vi "FRA_sensors_main.vi"() -> ()   [LabVIEW 2013]
uses:
  subVIs/UDP_read_datagram.ctl
  subVIs/UI_states.ctl
  <vilib>/Utility/file.llb/Read From Spreadsheet File (string).vi
panel:
  out "ACK'd_clients addr":u32[](array[numeric]) format="%x"
  in  "Power all sensors":bool
  out "Number of clients":i32
  in  "OK Button":bool
  in  "Power A3.3":bool
  in  "Power A3.2":bool
  in  "Power A3.1":bool
  in  "Power A3.0":bool
  in  "Power A2.3":bool
  in  "Power A2.2":bool
  in  "Power A2.1":bool
  in  "Power A2.0":bool
  in  "Power A1.3":bool
  in  "Power A1.2":bool
  in  "Power A1.1":bool
  in  "Power A1.0":bool
  out "Error message":string
  in  "listen on port":u16=1100
  out "data received":string
  in  "Stop Button":bool
  out "Datagram to send":string
  out "ACK'd_clients":u8[](array[numeric])
  # "OFF"
  # "ON"
  # "variables and settings"
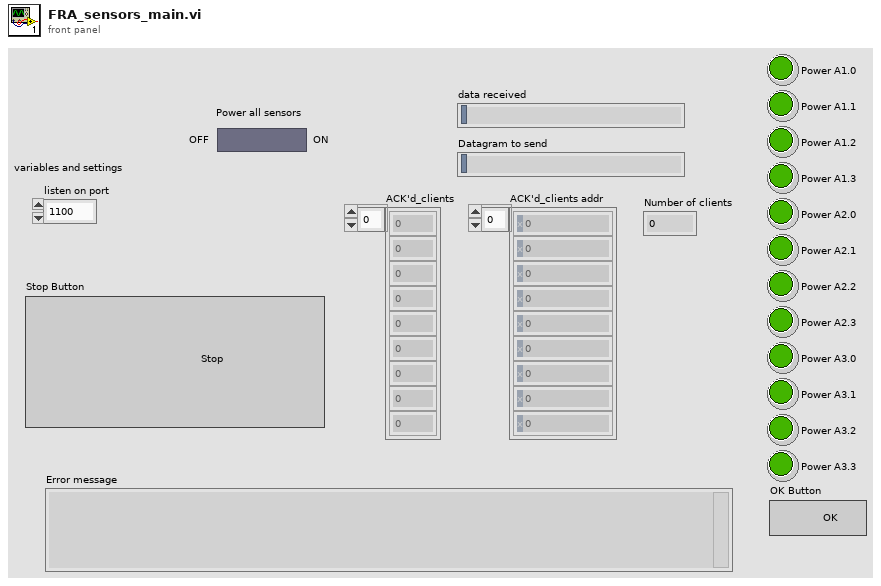
[diagram p1: front panel]
types:
  T1 = typedef "UI_states.ctl" = enum16{"SENS_PWR_CHANGE", "INIT", "IDLE", "RUN", "STOP", ""}
  T2 = typedef "UDP_read_datagram.ctl" = cluster{"msg":string, "address":u32, "port":u16}
  T3 = enum8{"Enabled", "Disabled", "Disabled and Grayed Out"}
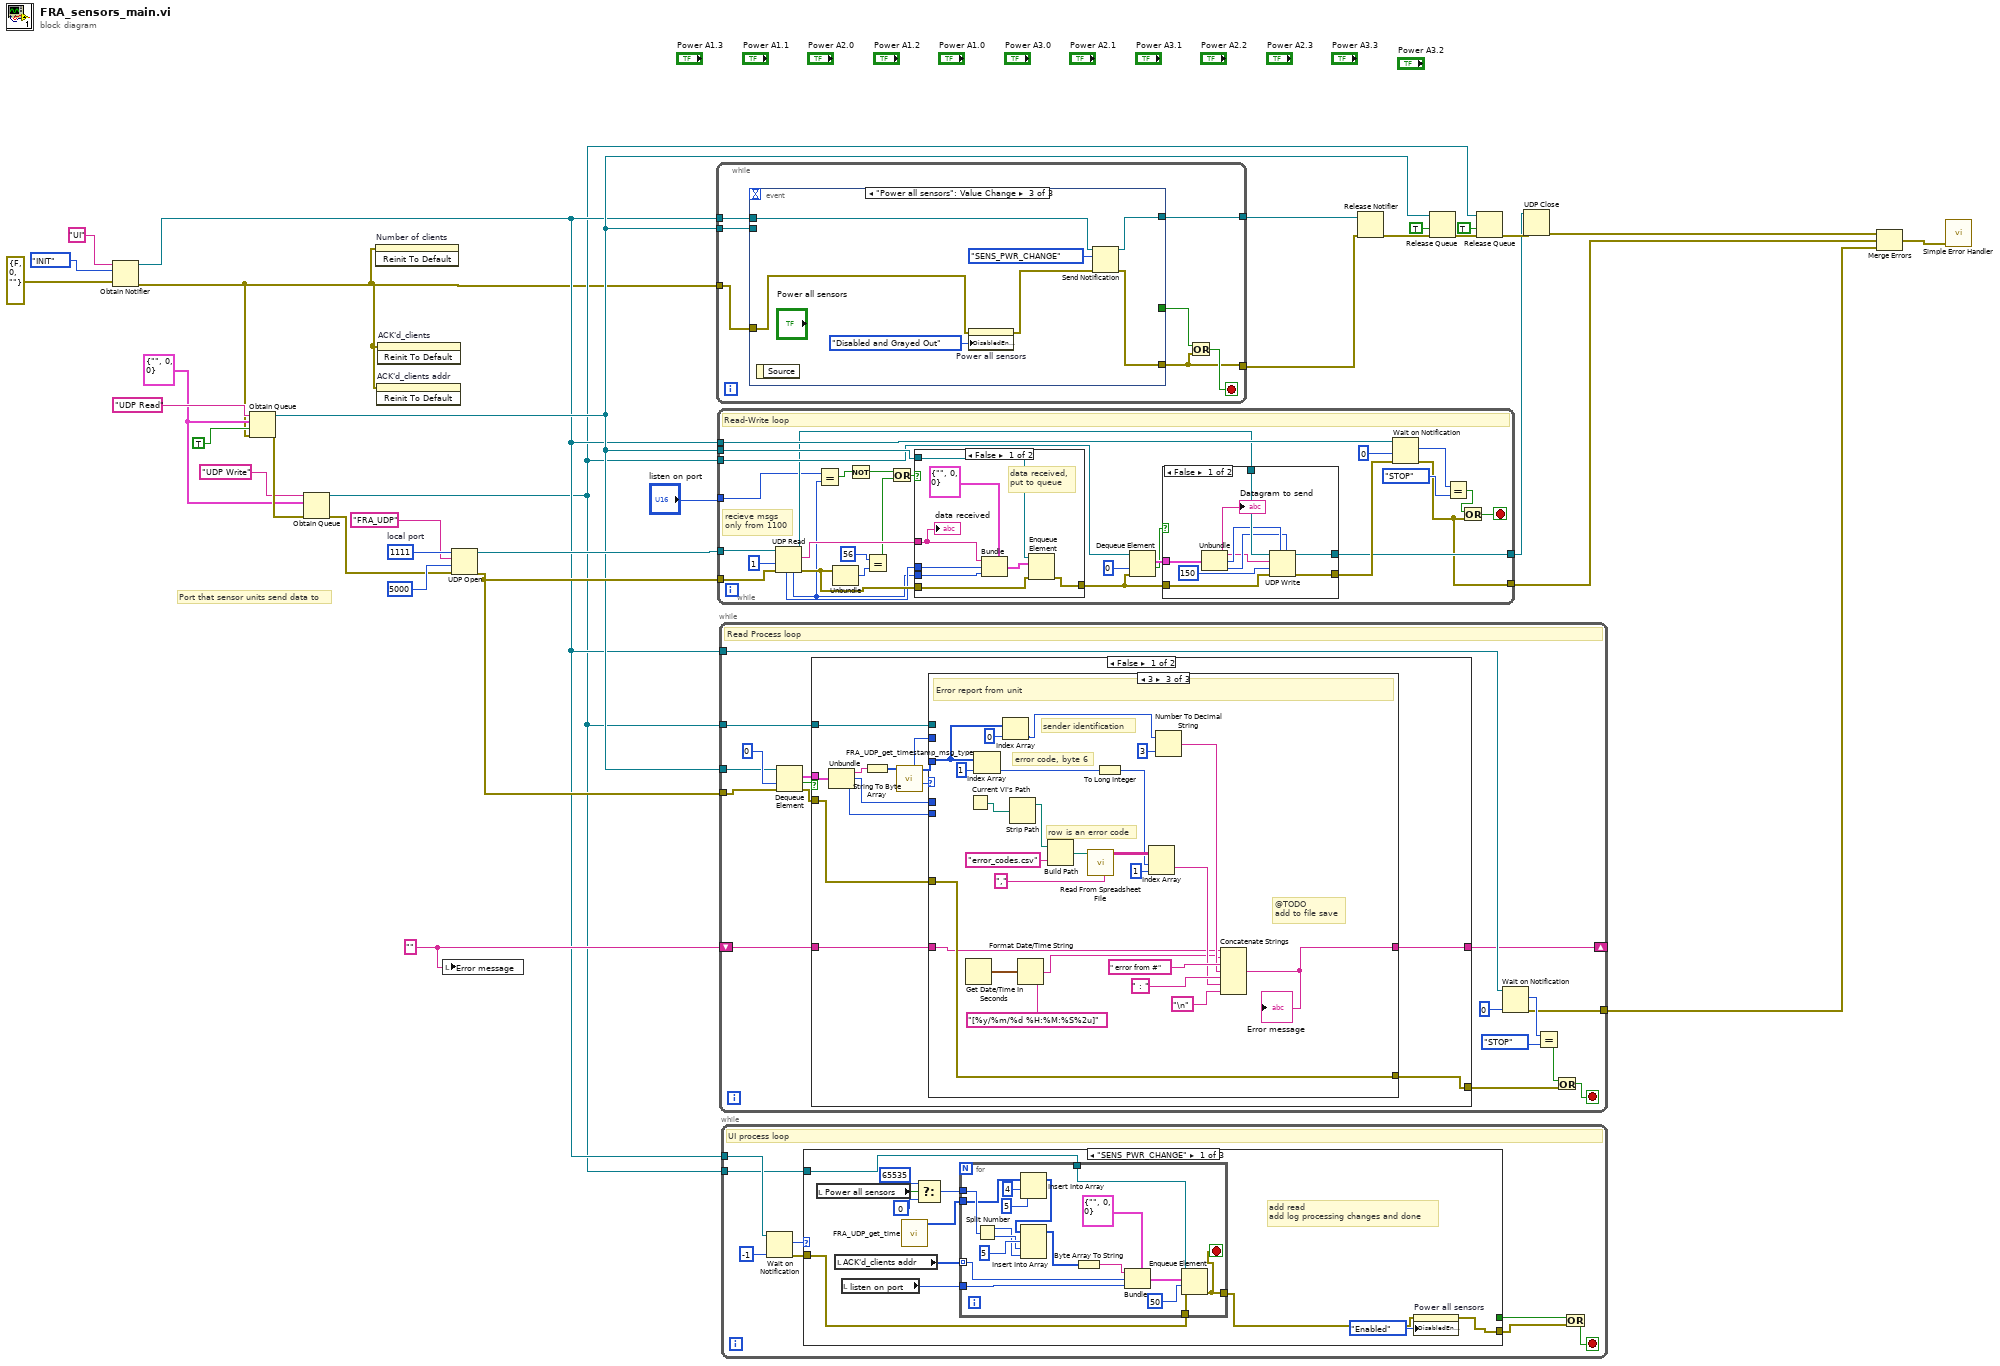
[diagram p0: block diagram]
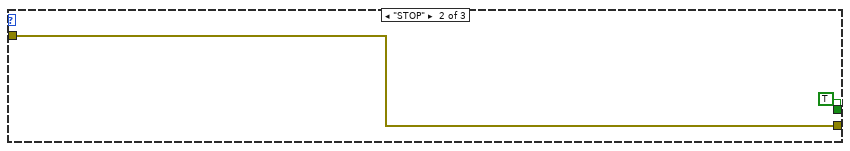
[diagram p2: hidden frame]
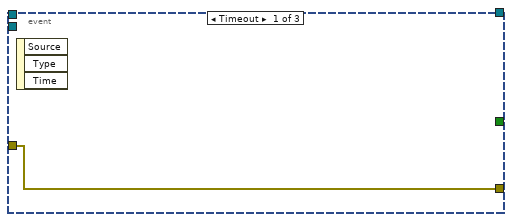
[diagram p4: hidden frame]
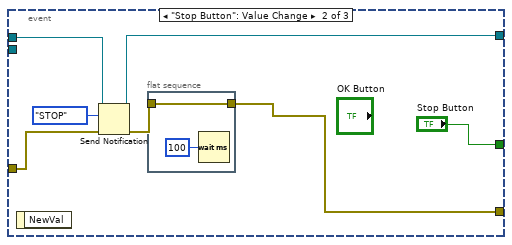
[diagram p5: hidden frame]
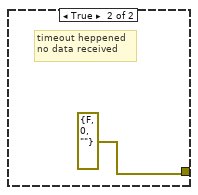
[diagram p7: hidden frame]
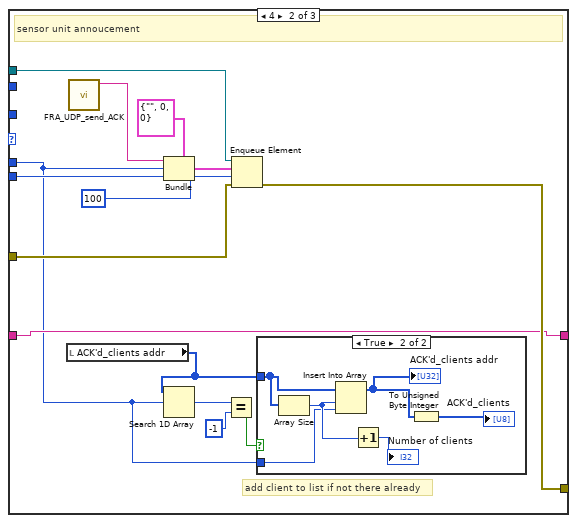
[diagram p9: hidden frame]
diagram:
  w4 = ""
  w13 = T2 {"msg"="", "address"=0, "port"=0}
  w32 = u16 1111  # local port
  # "Port that sensor units send data to"
  n1 = Obtain Notifier(name (unnamed)="UI", notification data type=UI_states."INIT" ("Enum"), error in (no error)=errorcluster {"status"=FALSE, "code"=0, "source"=""}) -> (notifier out=w3:refnum<notifier>, error out=w1:errorcluster)  [unwired: 1 in, 1 out]
  n2 = Obtain Queue(name (unnamed)="UDP Read", element data type=w13, create if not found? (T)=TRUE, error in (no error)=w1) -> (queue out=w9:refnum<queue>, error out=w15:errorcluster)  [unwired: 1 in, 1 out]
  n3 = Obtain Queue(name (unnamed)="UDP Write", element data type=w13, error in (no error)=w15) -> (queue out=w2:refnum<queue>, error out=w12:errorcluster)  [unwired: 2 in, 1 out]
  n4 = invoke on="Number of clients" class="DigNum (strict)" method="Reinit To Default"(error in=w1) -> ()  [unwired: 2 in, 3 out]
  n5 = invoke on="ACK'd_clients addr" class="Arr (strict)" method="Reinit To Default"(error in=w1) -> ()  [unwired: 2 in, 3 out]
  n6 = invoke on="ACK'd_clients" class="Arr (strict)" method="Reinit To Default"(error in=w1) -> ()  [unwired: 2 in, 3 out]
  n7 = local write "Error message"(w4) -> ()
  n8 = UDP Open(8:w12, 9:5000 ("timeout ms (25000)"), 10:"FRA_UDP" ("service name"), 11:w32) -> (port=w26:refnum<k16>, 0:w27:errorcluster)  [unwired: 1 in, 1 out]
  n9 = while {
    tunnel: w3 -> [w39]
    tunnel: w1 -> [w38]
    tunnel: [w35] -> w22
    tunnel: [w34] -> w21
    tunnel: w9 -> [w33]
    stop <- w36 stop-if-true
    n10 = event shown="[2] \"Power all sensors\": Value Change" {
      selector: _ -> [_ _ _]
      dyn-events: _ -> [_ _ _]
      timeout: _ -> [_ _ _]
      tunnel: w39 -> [_ w46 w55]
      tunnel: [w40 w41 w50] -> w34
      tunnel: w38 -> [w40 w44 w52]
      tunnel: [_ "Stop Button" _] -> w37
      tunnel: [_ w43 w54] -> w35
      tunnel: w33 -> [_ _ _]
      event Timeout {
        n11 = event-data() -> ()  [unwired: 1 in, 3 out]
      }
      event "Stop Button": Value Change {
        n12 = event-data() -> ()  [unwired: 1 in, 1 out]
        n13 = Send Notification(notification=UI_states."STOP", notifier=w46, error in (no error)=w44) -> (notifier out=w43:refnum<notifier>, error out=w42:errorcluster)
        n14 = flat-sequence {
          tunnel: w42 -> [w48]
          tunnel: [w48] -> w41
          frame #0 {
            n15 = Wait (ms)(milliseconds to wait=u32 100) -> ()  [unwired: 1 out]
          }
        }
      }
      event "Power all sensors": Value Change {
        n16 = event-data() -> ()  [unwired: 1 in, 1 out]
        n17 = property on="Power all sensors" class="Bool (strict)"(error in=w52, "DisabledEnum"=T3."Disabled and Grayed Out" ("Disabled")) -> (error out=w51:errorcluster)  [unwired: 1 in, 1 out]
        n18 = Send Notification(notification=UI_states."SENS_PWR_CHANGE", notifier=w55, error in (no error)=w51) -> (notifier out=w54:refnum<notifier>, error out=w50:errorcluster)
      }
    }
    n19 = Or(x=w37, y=w34) -> (x .or. y?=w36:bool)
  }
  n20 = while {
    tunnel: w9 -> [w75]
    tunnel: w27 -> [w80]
    tunnel: w26 -> [w85]
    tunnel: w3 -> [w84]
    tunnel: w2 -> [w72]
    tunnel: [w61] -> w11
    tunnel: "listen on port" -> [w60]
    tunnel: [w57] -> w8
    stop <- w58 stop-if-true
    # "recieve msgs\nonly from 1100"
    # "Read-Write loop"
    n21 = UDP Read(connection ID=w85, timeout ms (25000)=1, 8:w80) -> (data out=w76:string, error out=w77:errorcluster, 3:w70:refnum<k16>, 4:w63:u16, 6:w74:u32)  [unwired: 1 out]
    n22 = Equal?(x=w60, y=w63) -> (x = y?=w65:bool)
    n23 = Unbundle(w77) -> ("code"=w79:i32)  [unwired: 2 out]
    n24 = Not(x=w65) -> (.not. x?=w64:bool)
    n25 = Equal?(x=56, y=w79) -> (x = y?=w66:bool)
    n26 = Or(x=w64, y=w66) -> (x .or. y?=w67:bool)
    n27 = case shown="False" w67 {
      tunnel: w77 -> [w105 _]
      tunnel: [w99 errorcluster {"status"=FALSE, "code"=0, "source"=""} ("error out")] -> w69
      tunnel: w76 -> [w102 _]
      tunnel: w75 -> [w98 _]
      tunnel: w74 -> [w101 _]
      tunnel: w63 -> [w100 _]
      frame False {
        # "data received, \nput to queue"
        n28 = Bundle(cluster=T2 {"msg"="", "address"=0, "port"=0}, "msg"=w102, "address"=w101, "port"=w100) -> (w104:T2)
        n29 = Enqueue Element(queue=w98, element=w104, error in (no error)=w105) -> (error out=w99:errorcluster)  [unwired: 1 in, 2 out]
        "data received" <- w102
      }
      frame True {
        # "timeout heppened\nno data received"
      }
    }
    n30 = Dequeue Element(queue=w72, timeout in ms (-1)=0, error in (no error)=w69) -> (element=w71:T2, timed out?=w62:bool)  [unwired: 2 out]
    n31 = case shown="False" w62 {
      tunnel: w71 -> [w95 _]
      tunnel: w70 -> [w94 w96]
      tunnel: w69 -> [w92 w97]
      tunnel: [w89 w97] -> w68
      tunnel: [w88 w96] -> w61
      frame False {
        n32 = Unbundle(w95) -> ("msg"=w87:string, "address"=w91:u32, "port"=w90:u16)
        "Datagram to send" <- w87
        n33 = UDP Write(address=w91, port or service name=w90, connection ID=w94, data in=w87, 8:w92, 9:150 ("timeout ms (25000)")) -> (error out=w89:errorcluster, 3:w88:refnum<k16>)
      }
      frame True {
        # "no message in send buffer"
      }
    }
    n34 = Wait on Notification(notifier=w84, timeout in ms (-1)=0, error in (no error)=w68) -> (notification=w82:T1, error out=w57:errorcluster)  [unwired: 1 in, 2 out]
    n35 = Equal?(x=w82, y=UI_states."STOP") -> (x = y?=w59:bool)
    n36 = Or(x=w59, y=w57) -> (x .or. y?=w58:bool)
  }
  n37 = while {
    tunnel: w27 -> [w122]
    tunnel: w9 -> [w121]
    tunnel: w3 -> [w111]
    tunnel: w2 -> [w109]
    tunnel: [w110] -> w7
    shift-right: [w107] -> _
    shift-left: w4 -> [w108]
    stop <- w116 stop-if-true
    # "Read Process loop"
    n38 = Dequeue Element(queue=w121, timeout in ms (-1)=0, error in (no error)=w122) -> (element=w118:T2, timed out?=w120:bool, error out=w119:errorcluster)  [unwired: 1 out]
    n39 = case shown="False" w120 {
      tunnel: w119 -> [w127 w185]
      tunnel: w118 -> [w134 _]
      tunnel: [w126 w185] -> w117
      tunnel: w109 -> [w129 _]
      tunnel: w108 -> [w125 w184]
      tunnel: [w124 w184] -> w107
      frame False {
        n40 = Unbundle(w134) -> ("msg"=w133:string, "address"=w130:u32, "port"=w128:u16)
        n41 = String To Byte Array(string=w133) -> (unsigned byte array=w136:u8[])
        n42 = call "FRA_UDP_get_timestamp_msg_type.vi"("incoming_UDP"=w136) -> ("MSG_type_byte"=w135:u8, "datagram_rest"=w132:u8[], "Datagram number"=w131:u32)  [unwired: 6 in, 2 out]
        n43 = case shown="3" w135 {
          tunnel: w132 -> [_ _ w160]
          tunnel: w131 -> [_ _ _]
          tunnel: w130 -> [_ w140 _]
          tunnel: w129 -> [_ w145 _]
          tunnel: w128 -> [_ w147 _]
          tunnel: w127 -> [w138 w143 w171]
          tunnel: [w138 w142 w171] -> w126
          tunnel: w125 -> [w137 w141 w166]
          tunnel: [w137 w141 w169] -> w124
          frame 0, Default {
          }
          frame 4 {
            # "add client to list if not there already"
            # "sensor unit annoucement"
            n44 = local read "ACK'd_clients addr"() -> (w139:u32[])
            n45 = call "FRA_UDP_send_ACK.vi"() -> ("Datagram to send"=w148:string)  [unwired: 11 in]
            n46 = Bundle(cluster=T2 {"msg"="", "address"=0, "port"=0}, "msg"=w148, "address"=w140, "port"=w147) -> (w146:T2)
            n47 = Search 1D Array(1D array=w139, element=w140) -> (index of element=w152:i32)  [unwired: 1 in]
            n48 = Equal?(x=w152, y=-1) -> (x = y?=w150:bool)
            n49 = Enqueue Element(queue=w145, element=w146, timeout in ms (-1)=100, error in (no error)=w143) -> (error out=w142:errorcluster)  [unwired: 2 out]
            n50 = case shown="True" w150 {
              tunnel: w139 -> [_ w158]
              tunnel: w140 -> [_ w156]
              frame False {
              }
              frame True {
                n51 = Array Size(array=w158) -> (size(s)=w157:i32)
                n52 = Insert Into Array(array=w158, index=w157, new element=w156) -> (w153:u32[])
                "ACK'd_clients addr" <- w153
                n53 = Increment(x=w157) -> (x+1=→"Number of clients":i32)
                n54 = To Unsigned Byte Integer(number=w153) -> (unsigned 8bit integer=→"ACK'd_clients":u8[])
              }
            }
          }
          frame 3 {
            # "sender identification"
            # "error code, byte 6"
            # "@TODO\nadd to file save"
            # "row is an error code"
            # "Error report from unit"
            n55 = Get Date/Time In Seconds() -> (seconds since 1Jan1904=w165:timestamp)
            n56 = Current VI's Path() -> (path=w168:path)
            n57 = Index Array(array=w160, index=1) -> (element=w177:u8)
            n58 = Index Array(array=w160, index=0) -> (element=w159:u8)
            n59 = Strip Path(path=w168) -> (stripped path=w167:path)  [unwired: 1 out]
            n60 = Format Date/Time String(time format string (%c)="[%y/%m/%d %H:%M:%S%2u]", seconds (now)=w165) -> (date/time string=w164:string)  [unwired: 1 in]
            n61 = Build Path(base path=w167, name or relative path="error_codes.csv") -> (appended path=w182:path)
            n62 = call-poly <vilib>:"Read From Spreadsheet File.vi"("delimiter (\\t)"="," ("delimiter (\\t)"), "file path (dialog if empty)"=w182) -> ("all rows"=w179:string[][])  [unwired: 5 in, 4 out]
            n63 = To Long Integer(number=w177) -> (32bit integer=w176:i32)
            n64 = Index Array(array=w179, index (row)=w176, index (col)=1 ("disabled index (col)")) -> (element=w172:string)
            n65 = Number To Decimal String(number=w159, width (-)=i16 3) -> (decimal integer string=w174:string)
            n66 = Concatenate Strings(w166, w164, " error from #" ("string"), w174, " : " ("string"), w172, "\n" ("string")) -> (w169:string)
            "Error message" <- w169
          }
        }
      }
      frame True {
        # "dequeue timed out\nno message to read"
      }
    }
    n67 = Wait on Notification(notifier=w111, timeout in ms (-1)=0) -> (notification=w114:T1, error out=w110:errorcluster)  [unwired: 2 in, 2 out]
    n68 = Equal?(x=w114, y=UI_states."STOP") -> (x = y?=w112:bool)
    n69 = Or(x=w112, y=w117) -> (x .or. y?=w116:bool)
  }
  n70 = while {
    tunnel: w3 -> [w191]
    tunnel: w2 -> [w187]
    stop <- w192 stop-if-true
    # "UI process loop"
    n71 = Wait on Notification(notifier=w191, timeout in ms (-1)=-1) -> (notification=w190:T1, error out=w188:errorcluster)  [unwired: 2 in, 2 out]
    n72 = case shown="\"SENS_PWR_CHANGE\"" w190 {
      tunnel: [_ TRUE _] -> w189
      tunnel: [w197 w224 w226] -> w186
      tunnel: w188 -> [w195 w224 w226]
      tunnel: w187 -> [w200 _ _]
      frame "SENS_PWR_CHANGE" {
        # "add read\nadd log processing changes and done"
        n73 = local read "Power all sensors"() -> (w205:bool)
        n74 = local read "ACK'd_clients addr"() -> (w202:u32[])
        n75 = local read "listen on port"() -> (w199:u16)
        n76 = call "FRA_UDP_get_time.vi"() -> ("array"=w198:u8[])  [unwired: 10 in, 1 out]
        n77 = Select(t=u16 65535, s=w205, f=u16 0 ("t")) -> (s? t:f=w201:u16)
        n78 = for {
          tunnel: w202 -> [w219] mode=indexing
          tunnel: w201 -> [w216]
          tunnel: w200 -> [w220]
          tunnel: w199 -> [w218]
          tunnel: w198 -> [w215]
          tunnel: w195 -> [w207]
          tunnel: [w206] -> w194
          stop <- w206 stop-if-true
          n79 = Split Number(x=w216) -> (hi(x)=w208:u8, lo(x)=w210:u8)
          n80 = Insert Into Array(array=w215, index=4, new element=u8 5 ("new element/subarray")) -> (w212:u8[])
          n81 = Insert Into Array(array=w212, index=5, new element #1=w210, new element #2=w208) -> (w209:u8[])
          n82 = Byte Array To String(unsigned byte array=w209) -> (string=w217:string)
          n83 = Bundle(cluster=T2 {"msg"="", "address"=0, "port"=0}, "msg"=w217, "address"=w219, "port"=w218) -> (w223:T2)
          n84 = Enqueue Element(queue=w220, element=w223, timeout in ms (-1)=50, error in (no error)=w207) -> (error out=w206:errorcluster)  [unwired: 2 out]
        }
        n85 = property on="Power all sensors" class="Bool (strict)"(error in=w194, "DisabledEnum"=T3."Enabled" ("Disabled")) -> (error out=w197:errorcluster)  [unwired: 1 in, 1 out]
      }
      frame "STOP" {
      }
      frame Default {
      }
    }
    n86 = Or(x=w189, y=w186) -> (x .or. y?=w192:bool)
  }
  n87 = Release Notifier(notifier=w22, error in (no error)=w21) -> (error out=w19:errorcluster)  [unwired: 1 in, 2 out]
  n88 = Release Queue(queue=w9, force destroy? (F)=TRUE, error in (no error)=w19) -> (error out=w18:errorcluster)  [unwired: 2 out]
  n89 = Release Queue(queue=w2, force destroy? (F)=TRUE, error in (no error)=w18) -> (error out=w17:errorcluster)  [unwired: 2 out]
  n90 = UDP Close(connection ID=w11, 8:w17) -> (error out=w16:errorcluster)  [unwired: 1 out]
  n91 = Merge Errors(w16, w8, w7) -> (w20:errorcluster)
  n92 = call <vilib>:"Simple Error Handler.vi"("error in (no error)"=w20) -> ()  [unwired: 4 in, 5 out]
